vi "Pivot Module.vi"(5 "Boolean":bool=TRUE, 6 "Calibration Angle":dbl, 7 "Encoder Refnum":string="My AnalogChannel RefNum", 8 "Motor Speed":dbl, 9 "Motor Angle":dbl, 10 "Drive Motor Refnum":string="My Motor RefNum", 11 "Rotational Motor Refnum":string="My Motor RefNum") -> ()   [LabVIEW 2012]
uses:
  <vilib>/Rock Robotics/WPI/SafetyOutput/WPI_SafetyOutputConfigMenu.ctl
  Begin/Global Variables.vi
panel:
  in  "Drive Motor Refnum":string="My Motor RefNum"
  in  "Rotational Motor Refnum":string="My Motor RefNum"
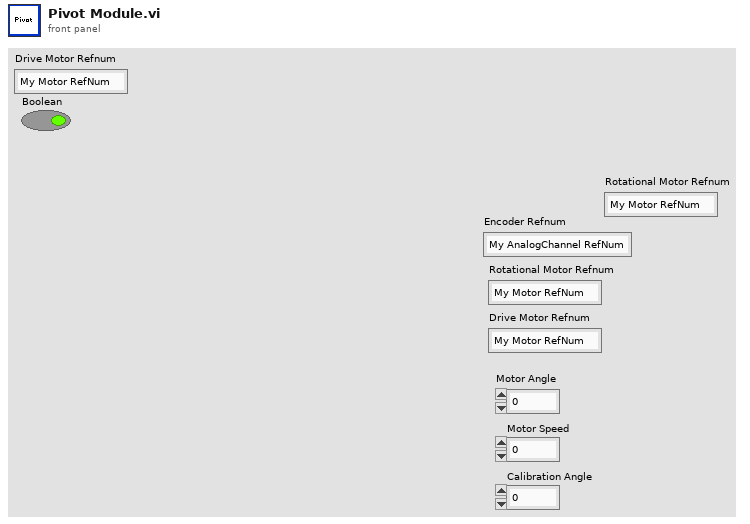
[diagram p1: front panel]
types:
  T1 = typedef "WPI_MotorControlDeviceRef.ctl" = cluster{"DeviceStatus":errorcluster, "Type":enum16{"PWM", "CAN"}, "PWM":cluster{"Digital Module":T2, "PWM Channel":T3, "DeadBand":T4}, "CAN":cluster{"Device Number":u8, "Control Mode":T5, "Semaphore":T6, "Max Vout":dbl}, "Invert":bool, "TransformRef":T7, "InvTransformRef":T7}
  T2 = typedef "FPGA_TypedefDigitalModule.ctl" = enum16{"Digital Module 1", "Digital Module 2"}
  T3 = typedef "FPGA_DIOPWMChannel.ctl" = enum8{"PWM 1", "PWM 2", "PWM 3", "PWM 4", "PWM 5", "PWM 6", "PWM 7", "PWM 8", "PWM 9", "PWM 10", "Invalid"}
  T4 = typedef "WPI_PWMDeadband.ctl" = cluster{"Name":string, "maxPositivePwm":i32, "minPositivePwm":i32, "centerPwm":i32, "maxNegativePwm":i32, "minNegativePwm":i32, "angularRange":u16}
  T5 = typedef "WPI_CANJaguar_ControlMode.ctl" = enum8{"Percent VBus", "Current", "Speed", "Position", "Voltage"}
  T6 = typedef "Semaphore RefNum" = refnum<k1>
  T7 = typedef "WPI_PWMTransform_ConPane.ctl" = refnum<vi>
  T8 = typedef "WPI_SafetyOutputConfigMenu.ctl" = enum16{"Enable", "Disable"}
  T9 = typedef "WPI_AnalogChannelDevRef.ctl" = cluster{"DevStatus":errorcluster, "Analog Module":T10, "Analog Channel":T11}
  T10 = typedef "FPGA_TypedefAnalogModule.ctl" = enum16{"Analog Module 1", "Analog Module 2"}
  T11 = typedef "FPGA_AIChannel.ctl" = enum8{"AI 1", "AI 2", "AI 3", "AI 4", "AI 5", "AI 6", "AI 7", "AI 8", "Invalid"}
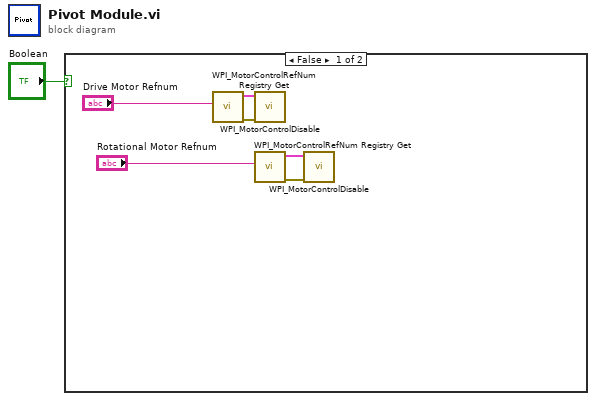
[diagram p0: block diagram]
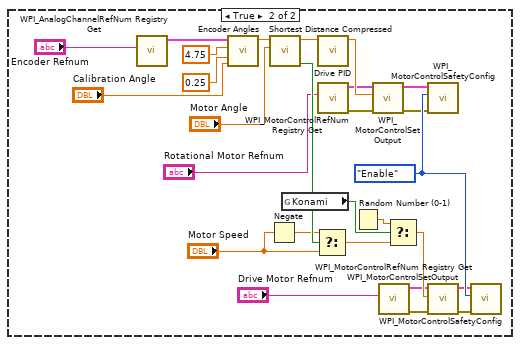
[diagram p2: hidden frame]
diagram:
  n1 = case shown="False" "Boolean" {
    frame False {
      n2 = call <vilib>:"WPI_MotorControlRefNum Registry Get.vi"("refnum name"="Drive Motor Refnum") -> ("error out"=w3:errorcluster, "MotorControlDevRef"=w4:T1)  [unwired: 9 in]
      n3 = call <vilib>:"WPI_MotorControlDisable.vi"("error in (no error)"=w3, "MotorControlDevRef"=w4) -> ()  [unwired: 8 in, 2 out]
      n4 = call <vilib>:"WPI_MotorControlRefNum Registry Get.vi"("refnum name"="Rotational Motor Refnum") -> ("error out"=w5:errorcluster, "MotorControlDevRef"=w6:T1)  [unwired: 9 in]
      n5 = call <vilib>:"WPI_MotorControlDisable.vi"("error in (no error)"=w5, "MotorControlDevRef"=w6) -> ()  [unwired: 8 in, 2 out]
    }
    frame True {
      w30 = WPI_SafetyOutputConfigMenu."Enable" ("mode")
      n6 = call <vilib>:"WPI_AnalogChannelRefNum Registry Get.vi"("refnum name"="Encoder Refnum") -> ("AIDeviceRef"=w9:T9)  [unwired: 9 in, 1 out]
      n7 = call "Encoder Angles.vi"("Calibration Angle"="Calibration Angle", "Bottom Voltage"=0.25, "Top Voltage"=4.75, "AIDeviceRef Encoder"=w9) -> ("Encoder Angle"=w10:dbl)  [unwired: 7 in]
      n8 = Negate(x="Motor Speed") -> (-x=w22:dbl)
      n9 = call "Shortest Distance Compressed.vi"("Needed angle"="Motor Angle", "Current Angle"=w10) -> ("Flip Motors?"=w28:bool, "Degrees to travel"=w16:dbl)  [unwired: 8 in]
      n10 = global read "Global Variables.vi" "Konami"() -> (w32:bool)
      n11 = Select(t=w22, s=w28, f="Motor Speed") -> (s? t:f=w34:dbl)
      n12 = call "Drive PID.vi"("Process Variable"=w16) -> ("Output"=w17:dbl)  [unwired: 10 in]
      n13 = call <vilib>:"WPI_MotorControlRefNum Registry Get.vi"("refnum name"="Rotational Motor Refnum") -> ("error out"=w12:errorcluster, "MotorControlDevRef"=w13:T1)  [unwired: 9 in]
      n14 = Random Number (0-1)() -> (number: 0 to 1=w31:dbl)
      n15 = call <vilib>:"WPI_MotorControlSetOutput.vi"("error in (no error)"=w12, "Output"=w17, "MotorControlDevRef"=w13) -> ("error out"=w15:errorcluster, "MotorControlDevRef"=w14:T1)  [unwired: 6 in, 1 out]
      n16 = call <vilib>:"WPI_MotorControlRefNum Registry Get.vi"("refnum name"="Drive Motor Refnum") -> ("error out"=w21:errorcluster, "MotorControlDevRef"=w20:T1)  [unwired: 9 in]
      n17 = Select(t=w31, s=w32, f=w34) -> (s? t:f=w33:dbl)
      n18 = call <vilib>:"WPI_MotorControlSafetyConfig.vi"("error in (no error)"=w15, "mode"=w30, "MotorControlDevRef"=w14) -> ()  [unwired: 7 in, 2 out]
      n19 = call <vilib>:"WPI_MotorControlSetOutput.vi"("error in (no error)"=w21, "Output"=w33, "MotorControlDevRef"=w20) -> ("error out"=w18:errorcluster, "MotorControlDevRef"=w19:T1)  [unwired: 6 in, 1 out]
      n20 = call <vilib>:"WPI_MotorControlSafetyConfig.vi"("error in (no error)"=w18, "mode"=w30, "MotorControlDevRef"=w19) -> ()  [unwired: 7 in, 2 out]
    }
  }
